vi "TMCM1021_goRef.vi"(2 "错误输入":errorcluster caption="错误输入（无错误）", 3 "motor":u8(ring) items=["x", "y", "z"], 4 "执行？":bool, 5 "com in":refnum<visa-resource-name>) -> (0 "错误输出":errorcluster, 1 "com out":refnum<visa-resource-name>)   [LabVIEW 2018]
uses:
  module_param.vi
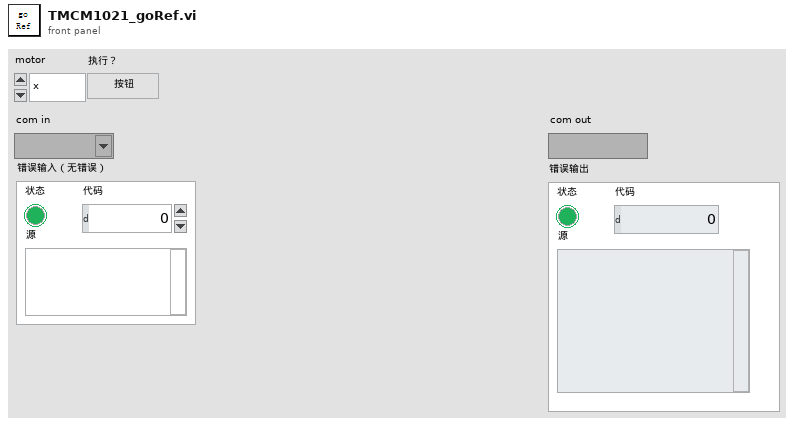
[diagram p1: front panel]
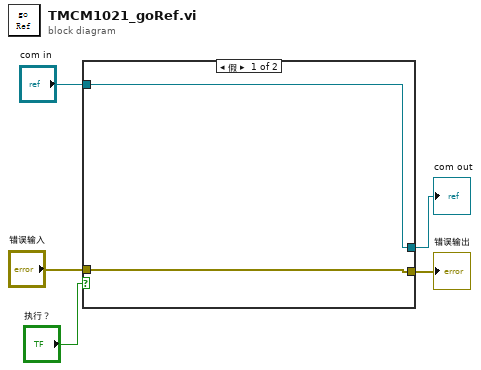
[diagram p0: block diagram]
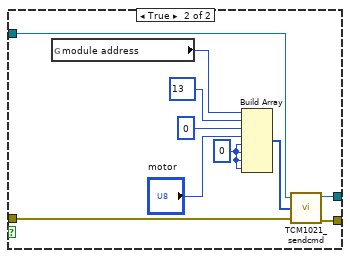
[diagram p2: hidden frame]
diagram:
  n1 = case shown="假" "执行？" {
    tunnel: "com in" -> [w7 w11]
    tunnel: "错误输入" -> [w6 w10]
    tunnel: [w7 w9] -> w2
    tunnel: [w6 w8] -> w1
    frame False {
    }
    frame True {
      w15 = u8 0 ("元素")
      n2 = global read "module_param.vi" "module address"() -> (w13:u8)
      n3 = Build Array(w13, u8 13, u8 0, "motor", w15, w15, w15, w15) -> (w12:u8[])
      n4 = call "TCM1021_sendcmd.vi"("com in"=w11, "command in"=w12, "错误输入"=w10) -> ("com out"=w9:refnum<visa-resource-name>, "错误输出"=w8:errorcluster)  [unwired: 2 out]
    }
  }
  "com out" <- w2
  "错误输出" <- w1
